vi "Format JSON Object.vi"(7 "Alphabetical Sort":bool, 8 "error in (no error)":errorcluster, 9 "Pretty Print?":bool, 10 "JSON elements":string[](array[string]), 11 "Names":string[](array[string])) -> (0 "error out":errorcluster, 3 "JSON Object Text out":string)   [LabVIEW 2020, in "JSONtext.lvlib"]
uses:
  <vilib>/JDP Science/JSONtext/JSONtext.lvlib
  <vilib>/JDP Science/JSONtext/support/quote and escape json string 2.vi
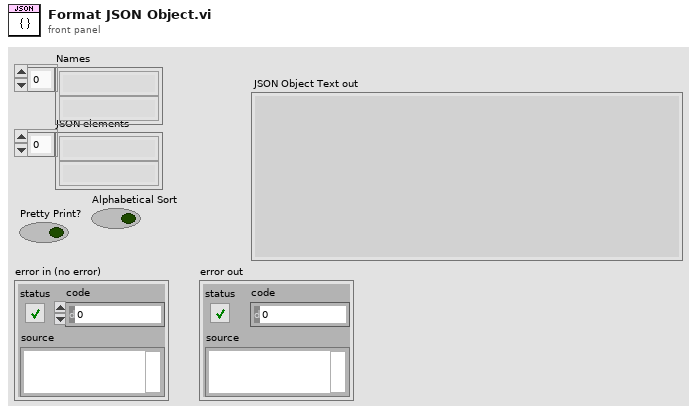
[diagram p1: front panel]
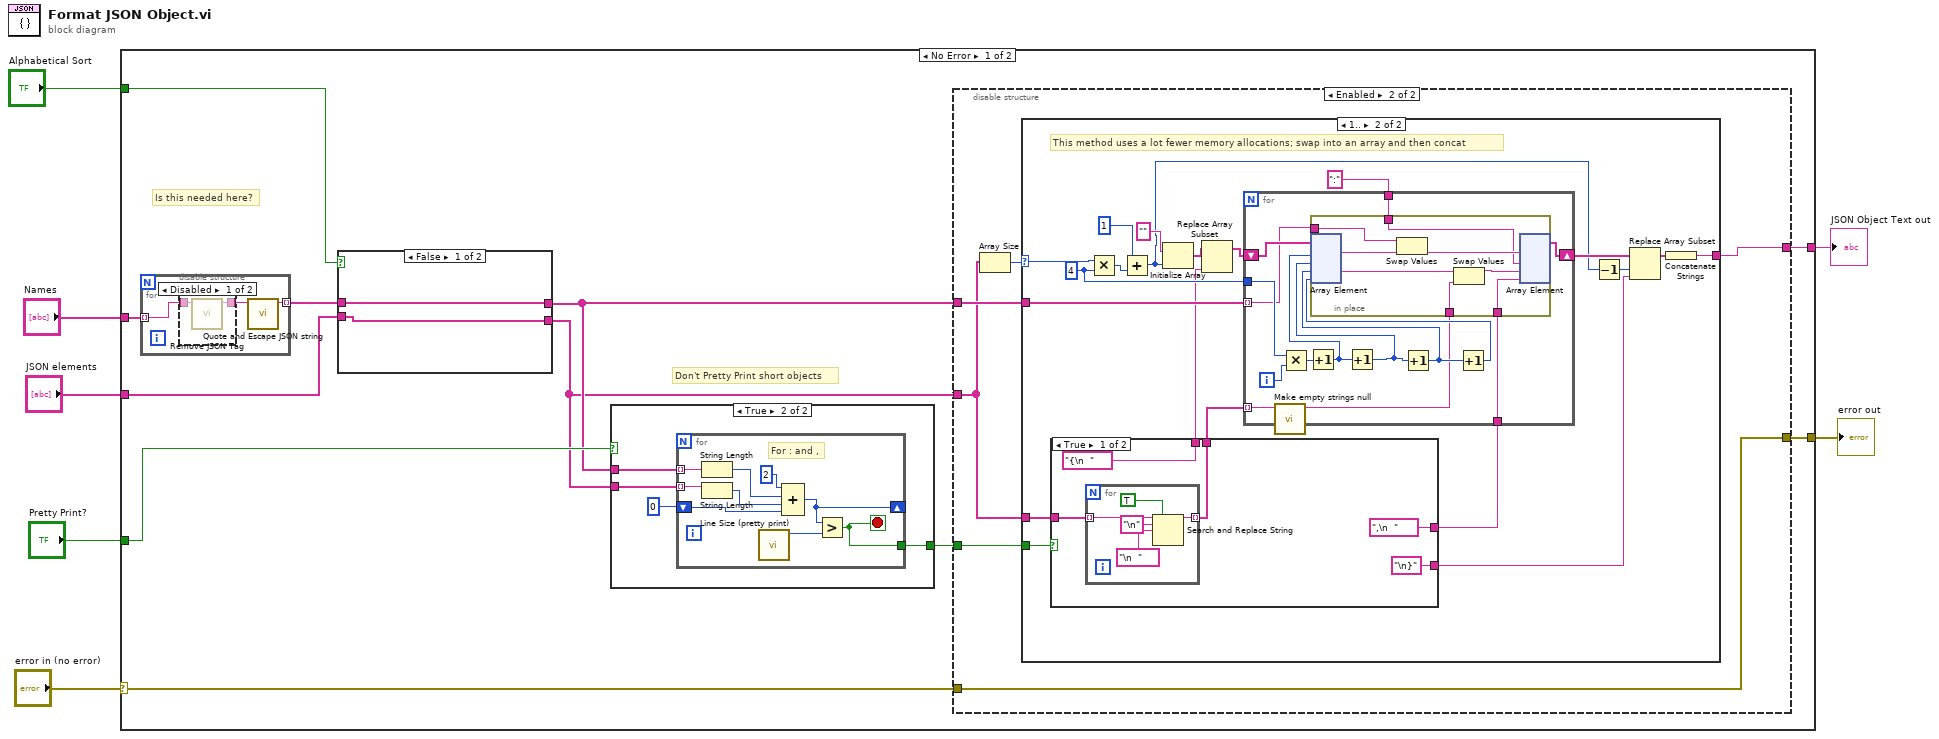
[diagram p0: block diagram]
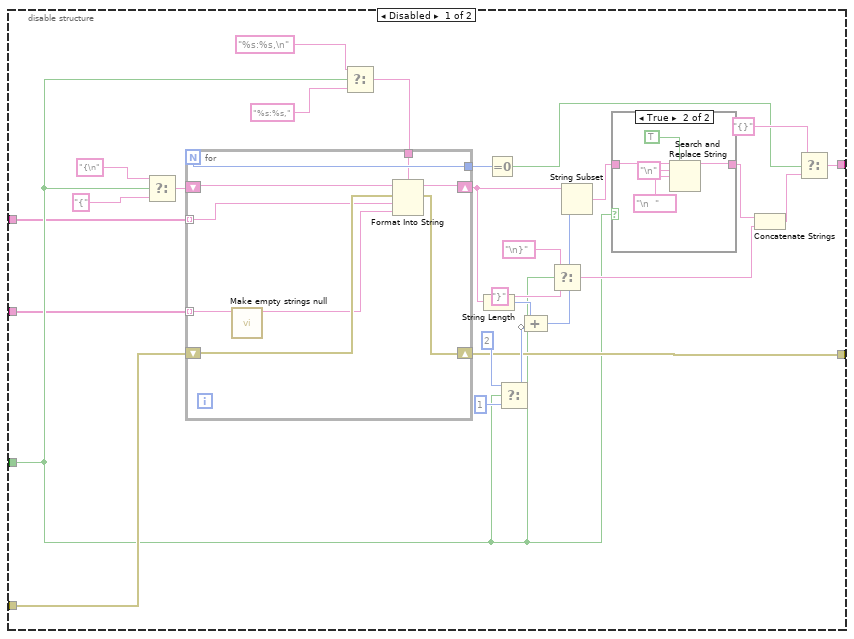
[diagram p2: hidden frame]
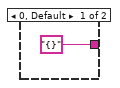
[diagram p4: hidden frame]
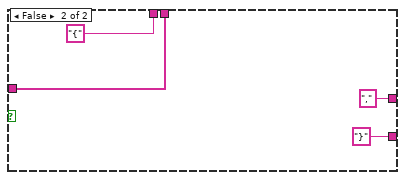
[diagram p5: hidden frame]
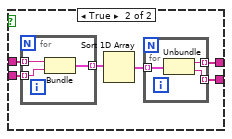
[diagram p6: hidden frame]
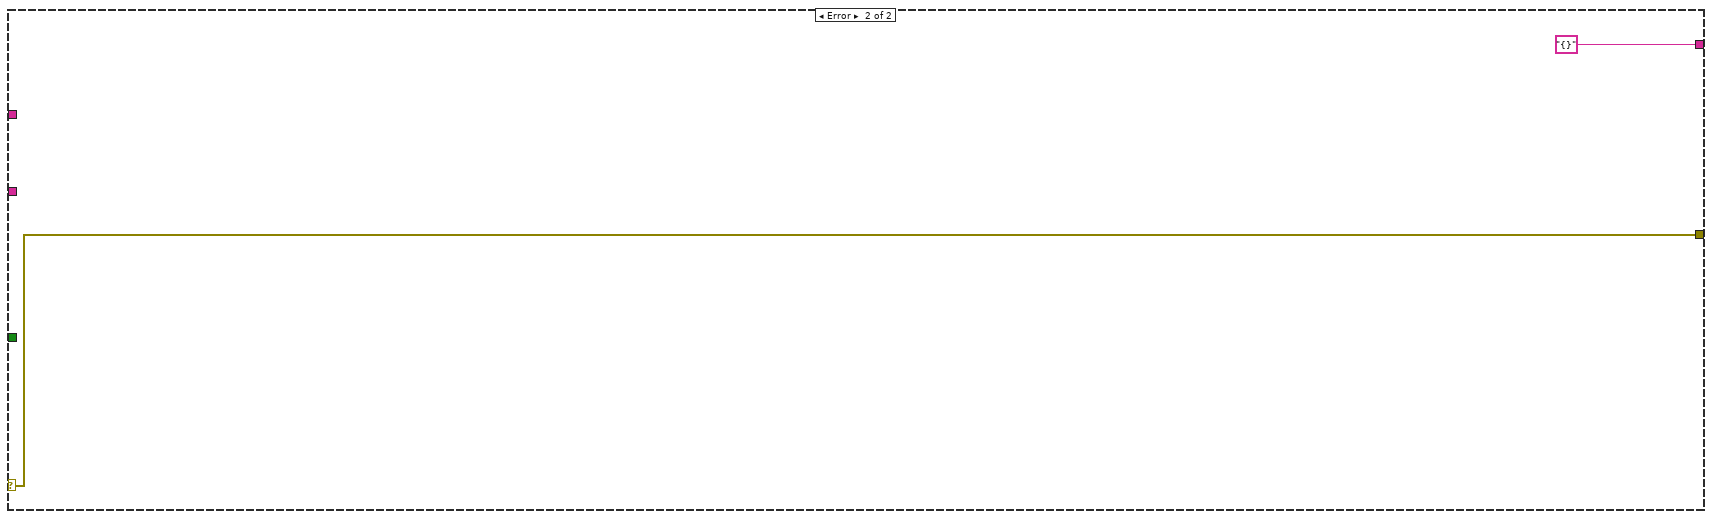
[diagram p9: hidden frame]
diagram:
  n1 = case shown="No Error" "error in (no error)" {
    selector: "error in (no error)" -> [w18 w158]
    tunnel: [w17 "{}" ("t")] -> w6
    tunnel: [w16 w158] -> w5
    tunnel: "Pretty Print?" -> [w15 _]
    tunnel: "Names" -> [w13 _]
    tunnel: "JSON elements" -> [w11 _]
    tunnel: "Alphabetical Sort" -> [w8 _]
    frame No Error {
      # "Is this needed here?"
      # "Don't Pretty Print short objects"
      n2 = for {
        tunnel: w13 -> [w139] mode=indexing
        tunnel: [w138] -> w12 mode=indexing
        n3 = disable-structure shown="Disabled" {
          disable-tunnel: [w142 w143] -> w140
          disable-tunnel: w139 -> [w141 w143]
          frame Disabled {
            n4 = call <vilib>:"Remove JSON Tag.vi"("Name"=w141) -> ("Name (tag stripped)"=w142:string)  [unwired: 9 in, 1 out]
          }
          frame Enabled {
          }
        }
        n5 = call <vilib>:"Quote and Escape JSON string.vi"("Plain Text"=w140) -> ("<JSON>"=w138:string)  [unwired: 10 in]
      }
      n6 = case shown="False" w8 {
        tunnel: w12 -> [w125 w131]
        tunnel: w11 -> [w124 w130]
        tunnel: [w125 w127] -> w10
        tunnel: [w124 w126] -> w9
        frame False {
        }
        frame True {
          n7 = for {
            tunnel: w131 -> [w137] mode=indexing
            tunnel: w130 -> [w136] mode=indexing
            tunnel: [w135] -> w129 mode=indexing
            n8 = Bundle("<JSON>"=w137, "String"=w136) -> (w135:cluster{"<JSON>":string, "String":string})  [unwired: 1 in]
          }
          n9 = Sort 1D Array(array=w129) -> (sorted array=w128:cluster{"<JSON>":string, "String":string}[])
          n10 = for {
            tunnel: w128 -> [w134] mode=indexing
            tunnel: [w133] -> w126 mode=indexing
            tunnel: [w132] -> w127 mode=indexing
            n11 = Unbundle(w134) -> ("<JSON>"=w132:string, "String"=w133:string)
          }
        }
      }
      n12 = case shown="True" w15 {
        tunnel: w9 -> [_ w147]
        tunnel: w10 -> [_ w146]
        tunnel: [_ w144] -> w14
        frame False {
        }
        frame True {
          n13 = for {
            tunnel: w147 -> [w155] mode=indexing
            tunnel: w146 -> [w156] mode=indexing
            shift-right: [w153] -> _
            shift-left: 0 -> [w154]
            tunnel: [w152] -> w144
            stop <- w152 stop-if-true
            # "For : and ,"
            n14 = String Length(string=w156) -> (length=w149:i32)
            n15 = String Length(string=w155) -> (length=w150:i32)
            n16 = call <vilib>:"Line Size (pretty print).vi"() -> ("Line Size"=w151:i32)  [unwired: 11 in]
            n17 = Compound Arithmetic op=ADD(2 ("value"), w149, w150, w154) -> (w153:i32)
            n18 = Greater?(x=w153, y=w151) -> (0:w152:bool)
          }
        }
      }
      n19 = disable-structure shown="Enabled" {
        disable-tunnel: w18 -> [w45 w63]
        disable-tunnel: [w38 w64] -> w17
        disable-tunnel: [w22 w63] -> w16
        disable-tunnel: w14 -> [w21 w62]
        disable-tunnel: w10 -> [w20 w65]
        disable-tunnel: w9 -> [w19 w61]
        frame Disabled {
          n20 = Select(t="{\n", s=w21, f="{") -> (s? t:f=w30:string)
          n21 = Select(t="%s:%s,\n" ("format string"), s=w21, f="%s:%s," ("format string")) -> (s? t:f=w41:string)
          n22 = for {
            N -> [w57]
            tunnel: w20 -> [w54] mode=indexing
            tunnel: w19 -> [w53] mode=indexing
            shift-right: [w58] -> w28
            shift-left: w30 -> [w60]
            shift-right: [w59] -> w22
            shift-left: w45 -> [w55]
            tunnel: [w57] -> w23
            tunnel: w41 -> [w56]
            n23 = call <vilib>:"Make empty strings null.vi"("JSON Input"=w53) -> ("<JSON>"=w52:string)  [unwired: 10 in]
            n24 = Format Into String(format string=w56, initial string=w60, error in=w55, w54, w52) -> (resulting string=w58:string, error out=w59:errorcluster)
          }
          n25 = String Length(string=w28) -> (length=w27:i32)
          n26 = Equal To 0?(x=w23) -> (x = 0?=w24:bool)
          n27 = Select(t=2, s=w21, f=1) -> (s? t:f=w44:i32)
          n28 = Compound Arithmetic op=ADD(w27, invert w44) -> (w29:i32)
          n29 = Select(t="\n}" ("substring (\"\")"), s=w21, f="}" ("substring (\"\")")) -> (s? t:f=w33:string)
          n30 = String Subset(string=w28, length (rest)=w29) -> (substring=w35:string)  [unwired: 1 in]
          n31 = case shown="True" w21 {
            tunnel: w35 -> [w46 w51]
            tunnel: [w46 w50] -> w36
            frame False {
            }
            frame True {
              n32 = Search and Replace String(replace all?=TRUE ("replace all? (F)"), input string=w51, search string="\n", replace string="\n  " ("search string")) -> (result string=w50:string)  [unwired: 4 in, 3 out]
            }
          }
          n33 = Concatenate Strings(w36, w33) -> (w37:string)
          n34 = Select(t="{}", s=w24, f=w37) -> (s? t:f=w38:string)
        }
        frame Enabled {
          n35 = Array Size(array=w61) -> (size(s)=w66:i32)
          n36 = case shown="1.." w66 {
            selector: w66 -> [_ w87]
            tunnel: w65 -> [_ w84]
            tunnel: ["{}" ("t") w79] -> w64
            tunnel: w62 -> [_ w72]
            tunnel: w61 -> [_ w70]
            frame 0, Default {
            }
            frame 1.. {
              w83 = 4 ("y")
              # "This method uses a lot fewer memory allocations; swap into an array and then concat"
              n37 = case shown="True" w72 {
                tunnel: [",\n  " ("new element/subarray") "," ("new element/subarray")] -> w81
                tunnel: ["\n}" ("new element/subarray") "}" ("new element/subarray")] -> w71
                tunnel: w70 -> [w90 w99]
                tunnel: [w89 w99] -> w69
                tunnel: ["{\n  " ("new element/subarray") "{" ("new element/subarray")] -> w68
                frame True {
                  n38 = for {
                    tunnel: w90 -> [w94] mode=indexing
                    tunnel: [w93] -> w89 mode=indexing
                    n39 = Search and Replace String(replace all?=TRUE ("replace all? (F)"), input string=w94, search string="\n", replace string="\n  " ("search string")) -> (result string=w93:string)  [unwired: 4 in, 3 out]
                  }
                }
                frame False {
                }
              }
              n40 = Multiply(x=w87, y=w83) -> (x*y=w86:i32)
              n41 = Add(x=1, y=w86) -> (x+y=w73:i32)
              n42 = Initialize Array("", w73) -> (w77:string[])
              n43 = Replace Array Subset(array=w77, new element=w68) -> (w78:string[])  [unwired: 1 in]
              n44 = for {
                tunnel: w69 -> [w112] mode=indexing
                tunnel: w84 -> [w102] mode=indexing
                shift-right: [w103] -> w76
                shift-left: w78 -> [w111]
                tunnel: w83 -> [w114]
                tunnel: ":" ("new element/subarray") -> [w106]
                tunnel: w81 -> [w104]
                i -> [w115]
                n45 = call <vilib>:"Make empty strings null.vi"("JSON Input"=w112) -> ("<JSON>"=w105:string)  [unwired: 10 in]
                n46 = Multiply(x=w114, y=w115) -> (x*y=w113:i32)
                n47 = Increment(x=w113) -> (x+1=w110:i32)
                n48 = Increment(x=w110) -> (x+1=w109:i32)
                n49 = Increment(x=w109) -> (x+1=w108:i32)
                n50 = Increment(x=w108) -> (x+1=w107:i32)
                n51 = in-place {
                  in-place-border: w106 -> [w119]
                  in-place-border: w105 -> [w118]
                  in-place-border: w104 -> [w117]
                  in-place-border: w102 -> [w116]
                  n52 = in-place-array #1(w111, w110, w109, w108, w107) -> (w123:string, w121:string)  [unwired: 2 out]
                  n53 = Swap Values(12:w116, 14:w123) -> (3:w122:string)  [unwired: 1 in, 1 out]
                  n54 = Swap Values(12:w121, 14:w118) -> (1:w120:string)  [unwired: 1 in, 1 out]
                  n55 = in-place-array #1(w122, w119, w120, w117) -> (w103:string[])  [unwired: 4 out]
                }
              }
              n56 = Decrement(x=w73) -> (x-1=w74:i32)
              n57 = Replace Array Subset(array=w76, new element=w71, index=w74) -> (w75:string[])
              n58 = Concatenate Strings(w75) -> (w79:string)
            }
          }
        }
      }
    }
    frame Error {
    }
  }
  "JSON Object Text out" <- w6
  "error out" <- w5
